vi "(SubVI)I2C_Auto ID Scan.vi"(7 "Clock":T1=enum."400kHz", 8 "error in (no error)":errorcluster caption="에러 입력(에러 없음)") -> (0 "error out":errorcluster caption="에러 출력", 3 "ID found":u8[](array[numeric]))   [LabVIEW 2020]
uses:
  Controls/(Ctrl)I2C_Clock.ctl
  Serial/Controls/(Ctrl)Serial_Write Read Option.ctl
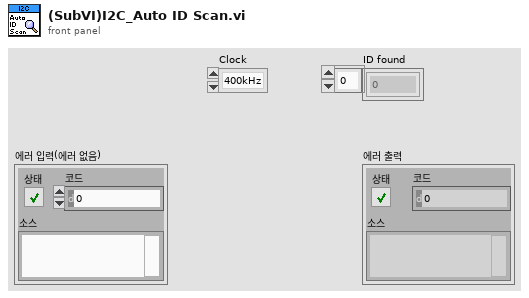
[diagram p1: front panel]
types:
  T1 = typedef "(Ctrl)I2C_Clock.ctl" = enum8{"1MHz", "2MHz", "3MHz", "400kHz"}
  T2 = typedef "(Ctrl)Serial_Write Read Option.ctl" = cluster{"Echo Request":bool, "Header Verification":bool, "Checksum Verification":bool, "User Code Verifiaction":bool}
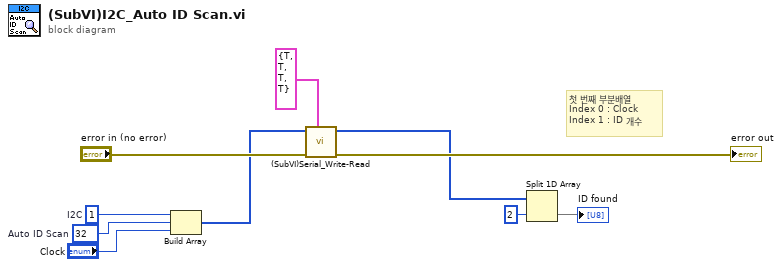
[diagram p0: block diagram]
diagram:
  w8 = u8 32  # Auto ID Scan
  w9 = u8 1  # I2C
  # "첫 번째 부분배열\nIndex 0 : Clock\nIndex 1 : ID 개수"
  n1 = Build Array(w9, w8, "Clock") -> (w2:u8[])
  n2 = call "(SubVI)Serial_Write-Read.vi"("Option"=T2 {"Echo Request"=TRUE, "Header Verification"=TRUE, "Checksum Verification"=TRUE, "User Code Verifiaction"=TRUE}, "error in (no error)"="error in (no error)", "Data to Write"=w2) -> ("error out"=→"error out":errorcluster, "Read Data"=w1:u8[])  [unwired: 6 in, 1 out]
  n3 = Split 1D Array(array=w1, index=2 ("인덱스")) -> (second subarray=→"ID found":u8[])  [unwired: 1 out]
